vi "AIDI-Initialize DI Clock Source.vi"(0 "Sync Task":refnum<k21>, 5 "DAQmx Device Name":tag="PXI1Slot4", 7 "Fs (Hz)":dbl, 11 "error in (no error)":errorcluster) -> (4 "clock task":refnum<k21>, 15 "error out":errorcluster)   [LabVIEW 2015]
uses:
  <vilib>/DAQmx/create/channels.llb/DAQmx Create Channel (CO-Pulse Generation-Ticks).vi
  <vilib>/DAQmx/configure/timing.llb/DAQmx Timing (Implicit).vi
  <vilib>/DAQmx/configure/trigger.llb/DAQmx Start Trigger (Digital Edge).vi
  <resource>/objmgr/daqmx.rc
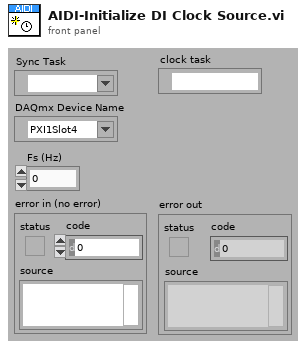
[diagram p1: front panel]
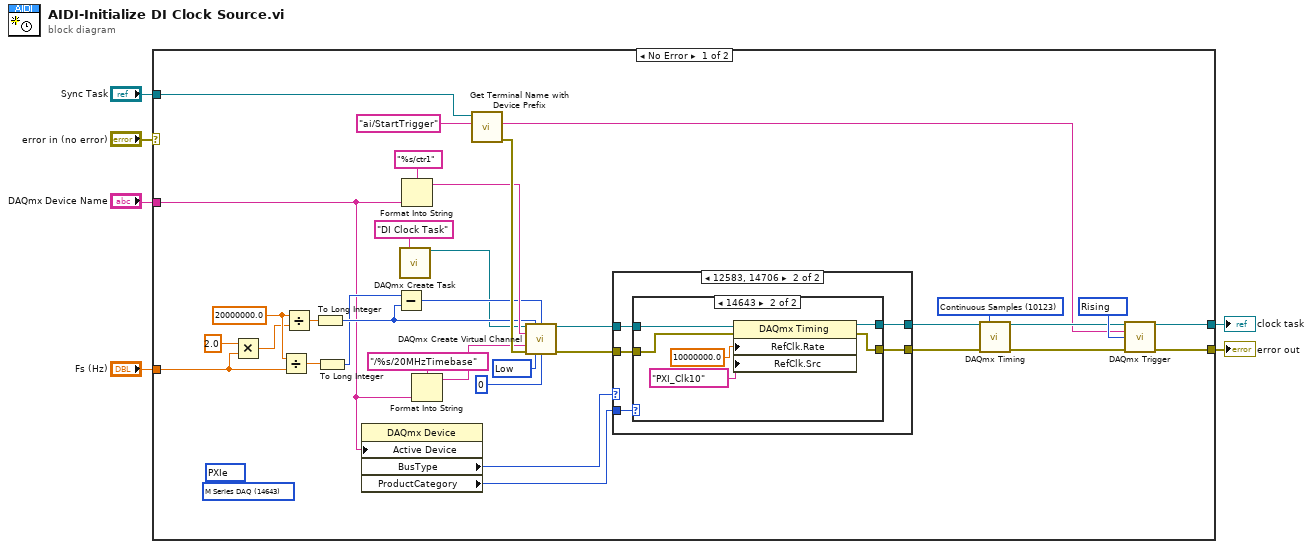
[diagram p0: block diagram]
diagram:
  n1 = case shown="No Error" "error in (no error)" {
    selector: "error in (no error)" -> [_ w56]
    tunnel: [w40 w56] -> w6
    tunnel: "DAQmx Device Name" -> [w15 _]
    tunnel: "Sync Task" -> [w14 _]
    tunnel: "Fs (Hz)" -> [w10 _]
    tunnel: [w13 _] -> w1
    frame No Error {
      (unwired) 14643 items=["M Series DAQ"=14643, "X Series DAQ"=15858, "E Series DAQ"=14642, "S Series DAQ"=14644, "B Series DAQ"=14662, "SC Series DAQ"=14645, "USB DAQ"=14646, "AO Series"=14647, "Digital I/O"=14648, "TIO Series"=14661, "Dynamic Signal Acquisition"=14649, "Switches"=14650, "CompactDAQ Chassis"=14658, "C Series Module"=14659, "SCXI Module"=14660, "SCC Connector Block"=14704, "SCC Module"=14705, "NI ELVIS"=14755, "Network DAQ"=14829, "SC Express"=15886, "Unknown"=12588] ("ProductCategory")
      (unwired) 14706 items=["PCI"=12582, "PCIe"=13612, "PXI"=12583, "PXIe"=14706, "SCXI"=12584, "SCC"=14707, "PCCard"=12585, "USB"=12586, "CompactDAQ"=14637, "TCP/IP"=14828, "Unknown"=12588, "SwitchBlock"=15870] ("BusType")
      w12 = 20000000.0 ("x")
      w24 = 10214 items=["High"=10192, "Low"=10214] ("idle state")
      w38 = 10280 items=["Rising"=10280, "Falling"=10171] ("Trigger Edge")
      w39 = 10123 items=["Finite Samples"=10178, "Continuous Samples"=10123] ("sample mode")
      n2 = Multiply(x=2.0, y=w10) -> (x*y=w11:dbl)
      n3 = Divide(x=w12, y=w10) -> (x/y=w22:dbl)
      n4 = Divide(x=w12, y=w11) -> (x/y=w23:dbl)
      n5 = To Long Integer(number=w23) -> (32bit integer=w21:i32)
      n6 = To Long Integer(number=w22) -> (32bit integer=w20:i32)
      n7 = property class="DAQmx Device"("Active Device"=w15) -> ("BusType"=w17:i32, "ProductCategory"=w16:i32)  [unwired: 2 in, 2 out]
      n8 = Subtract(x=w20, y=w21) -> (x-y=w19:i32)
      n9 = call <vilib>:"DAQmx Create Task.vi"("new task name"="DI Clock Task" ("name to assign")) -> ("task out"=w7:refnum<k21>)  [unwired: 13 in, 1 out]
      n10 = Format Into String(format string="%s/ctr1", w15) -> (resulting string=w26:string)  [unwired: 2 in, 1 out]
      n11 = Format Into String(format string="/%s/20MHzTimebase", w15) -> (resulting string=w18:string)  [unwired: 2 in, 1 out]
      n12 = call "Get Terminal Name with Device Prefix.vi"("Local Terminal Name"="ai/StartTrigger", "task/channels in"=w14) -> ("error out"=w31:errorcluster, "Terminal Name with Device Prefix"=w32:tag)  [unwired: 7 in, 1 out]
      n13 = call-poly <vilib>:"DAQmx Create Virtual Channel.vi"("task in"=w7, "high ticks"=w21, "low ticks"=w19, "counter"=w26, "source of ticks"=w18, "error in"=w31, "idle state"=w24, "initial delay"=u32 0) -> ("task out"=w29:refnum<k21>, "error out"=w30:errorcluster)  [unwired: 6 in]
      n14 = case shown="12583, 14706" w17 {
        tunnel: [w42 w47] -> w36
        tunnel: [w41 w46] -> w35
        tunnel: w30 -> [w41 w45]
        tunnel: w29 -> [w42 w44]
        tunnel: w16 -> [_ w43]
        frame 0, Default {
        }
        frame 12583, 14706 {
          n15 = case shown="14643" w43 {
            tunnel: [w49 w55] -> w47
            tunnel: [w48 w54] -> w46
            tunnel: w45 -> [w48 w53]
            tunnel: w44 -> [w49 w52]
            frame 0, Default {
            }
            frame 14643 {
              n16 = property class="DAQmx Timing"(reference=w52, error in=w53, "RefClk.Rate"=10000000.0, "RefClk.Src"=tag "PXI_Clk10") -> (reference out=w55:refnum<k21>, error out=w54:errorcluster)
            }
          }
        }
      }
      n17 = call-poly <vilib>:"DAQmx Timing.vi"("task/channels in"=w36, "sample mode"=w39, "error in"=w35) -> ("task out"=w34:refnum<k21>, "error out"=w33:errorcluster)  [unwired: 11 in]
      n18 = call-poly <vilib>:"DAQmx Trigger.vi"("task/channels in"=w34, "source"=w32, "edge"=w38, "error in"=w33) -> ("task out"=w13:refnum<k21>, "error out"=w40:errorcluster)  [unwired: 10 in]
    }
    frame Error {
    }
  }
  "error out" <- w6
  "clock task" <- w1
